vi "Draw Robot.vi"(7 "Gyro":dbl=-0.11, 10 "XY":cluster{"X":dbl, "Y":dbl}) -> (2 "Graph 2":cluster{cluster{"X":dbl, "Y":dbl}[]}[](graph)=[{[{"X"=44.0, "Y"=76.0}, {"X"=44.0, "Y"=76.0}]}, {[{"X"=30.03458329904793, "Y"=57.973155118857626}, {"X"=30.03458329904793, "Y"=57.973155118857626}]}, {[{"X"=29.965468303127132, "Y"=93.97308877320398}, {"X"=29.965468303127132, "Y"=93.97308877320398}]}, {[{"X"=57.96541670095207, "Y"=94.02684488114238}, {"X"=57.96541670095207, "Y"=94.02684488114238}]}, {[{"X"=58.03453169687287, "Y"=58.026911226796024}, {"X"=58.03453169687287, "Y"=58.026911226796024}]}, {[{"X"=43.942404170066, "Y"=105.9999447119553}, {"X"=43.942404170066, "Y"=105.9999447119553}]}])   [LabVIEW 2018]
panel:
  in  "Robot Lenght":dbl=44.0
  in  "Robot Width":dbl=28.0
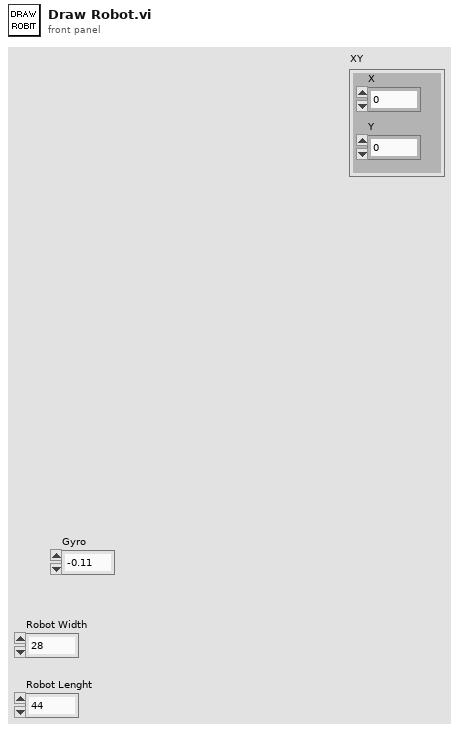
[diagram p1: front panel]
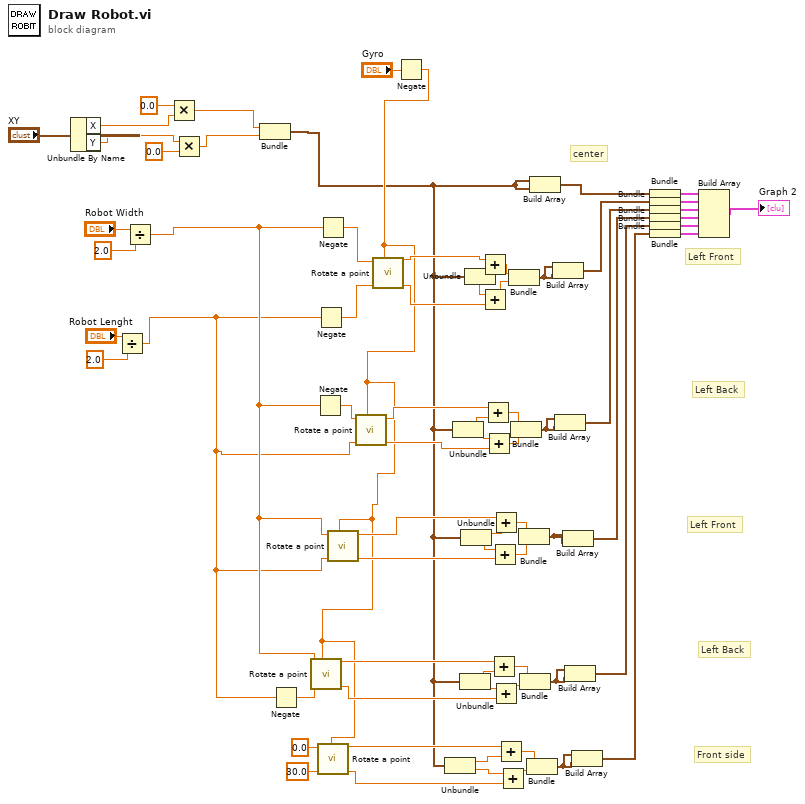
[diagram p0: block diagram]
diagram:
  # "center"
  # "Front side"
  # "Left Back"
  # "Left Front"
  # "Left Back"
  # "Left Front"
  n1 = Unbundle By Name("XY") -> ("X"=w6:dbl, "Y"=w4:dbl)
  n2 = Divide(x="Robot Lenght", y=2.0) -> (x/y=w50:dbl)
  n3 = Divide(x="Robot Width", y=2.0) -> (x/y=w51:dbl)
  n4 = Multiply(x=0.0, y=w6) -> (x*y=w5:dbl)
  n5 = Multiply(x=w4, y=0.0) -> (x*y=w3:dbl)
  n6 = Bundle(w5, w3) -> (w7:cluster{dbl, dbl})  [unwired: 1 in]
  n7 = Negate(x=w50) -> (-x=w55:dbl)
  n8 = Negate(x=w51) -> (-x=w52:dbl)
  n9 = Negate(x=w50) -> (-x=w53:dbl)
  n10 = Negate(x=w51) -> (-x=w54:dbl)
  n11 = Negate(x="Gyro") -> (-x=w9:dbl)
  n12 = call "Rotate a point.vi"("Gyro"=w9, "Y"=w55, "X"=w51) -> ("Y'"=w26:dbl, "X'"=w27:dbl)  [unwired: 7 in]
  n13 = call "Rotate a point.vi"("Gyro"=w9, "Y"=30.0, "X"=0.0) -> ("Y'"=w21:dbl, "X'"=w20:dbl)  [unwired: 7 in]
  n14 = call "Rotate a point.vi"("Gyro"=w9, "Y"=w50, "X"=w51) -> ("Y'"=w28:dbl, "X'"=w29:dbl)  [unwired: 7 in]
  n15 = call "Rotate a point.vi"("Gyro"=w9, "Y"=w50, "X"=w52) -> ("Y'"=w38:dbl, "X'"=w39:dbl)  [unwired: 7 in]
  n16 = call "Rotate a point.vi"("Gyro"=w9, "Y"=w53, "X"=w54) -> ("Y'"=w44:dbl, "X'"=w45:dbl)  [unwired: 7 in]
  n17 = Unbundle(w7) -> (w14:dbl, w13:dbl)
  n18 = Unbundle(w7) -> (w42:dbl, w41:dbl)
  n19 = Unbundle(w7) -> (w32:dbl, w30:dbl)
  n20 = Unbundle(w7) -> (w37:dbl, w34:dbl)
  n21 = Unbundle(w7) -> (w49:dbl, w48:dbl)
  n22 = Add(x=w45, y=w49) -> (x+y=w46:dbl)
  n23 = Add(x=w48, y=w44) -> (x+y=w47:dbl)
  n24 = Add(x=w39, y=w42) -> (x+y=w43:dbl)
  n25 = Add(x=w41, y=w38) -> (x+y=w40:dbl)
  n26 = Add(x=w27, y=w32) -> (x+y=w33:dbl)
  n27 = Add(x=w34, y=w28) -> (x+y=w36:dbl)
  n28 = Add(x=w29, y=w37) -> (x+y=w35:dbl)
  n29 = Add(x=w30, y=w26) -> (x+y=w31:dbl)
  n30 = Add(x=w20, y=w14) -> (x+y=w18:dbl)
  n31 = Add(x=w13, y=w21) -> (x+y=w19:dbl)
  n32 = Bundle(w46, w47) -> (w67:cluster{dbl, dbl})  [unwired: 1 in]
  n33 = Bundle(w43, w40) -> (w66:cluster{dbl, dbl})  [unwired: 1 in]
  n34 = Bundle(w35, w36) -> (w63:cluster{dbl, dbl})  [unwired: 1 in]
  n35 = Bundle(w33, w31) -> (w64:cluster{dbl, dbl})  [unwired: 1 in]
  n36 = Bundle(w18, w19) -> (w17:cluster{dbl, dbl})  [unwired: 1 in]
  n37 = Build Array(w7, w7) -> (w69:cluster{dbl, dbl}[])
  n38 = Build Array(w67, w67) -> (w68:cluster{dbl, dbl}[])
  n39 = Build Array(w66, w66) -> (w65:cluster{dbl, dbl}[])
  n40 = Build Array(w63, w63) -> (w62:cluster{dbl, dbl}[])
  n41 = Build Array(w64, w64) -> (w61:cluster{dbl, dbl}[])
  n42 = Build Array(w17, w17) -> (w15:cluster{dbl, dbl}[])
  n43 = Bundle(w69) -> (w70:cluster{cluster{dbl, dbl}[]})  [unwired: 1 in]
  n44 = Bundle(w68) -> (w25:cluster{cluster{dbl, dbl}[]})  [unwired: 1 in]
  n45 = Bundle(w65) -> (w24:cluster{cluster{dbl, dbl}[]})  [unwired: 1 in]
  n46 = Bundle(w62) -> (w23:cluster{cluster{dbl, dbl}[]})  [unwired: 1 in]
  n47 = Bundle(w61) -> (w22:cluster{cluster{dbl, dbl}[]})  [unwired: 1 in]
  n48 = Bundle(w15) -> (w16:cluster{cluster{dbl, dbl}[]})  [unwired: 1 in]
  n49 = Build Array(w70, w25, w24, w23, w22, w16) -> (→"Graph 2":cluster{cluster{dbl, dbl}[]}[])
